vi "SQL Open.vi"(8 "error in (no error)":errorcluster, 11 "Ini Reference":T1) -> (0 "error out":errorcluster, 3 "SQL Address":string)   [LabVIEW 2012]
uses:
  <vilib>/Utility/config.llb/Config Data RefNum.ctl
  <vilib>/Utility/config.llb/Read Key (String).vi
  <vilib>/Utility/config.llb/NI_LVConfig.lvlib
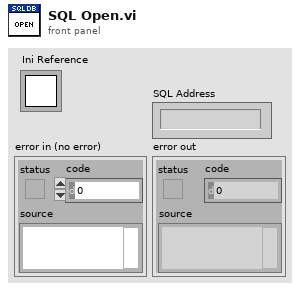
[diagram p1: front panel]
types:
  T1 = typedef "NI_LVConfig.lvlib/Config Data RefNum.ctl" = refnum<k1>
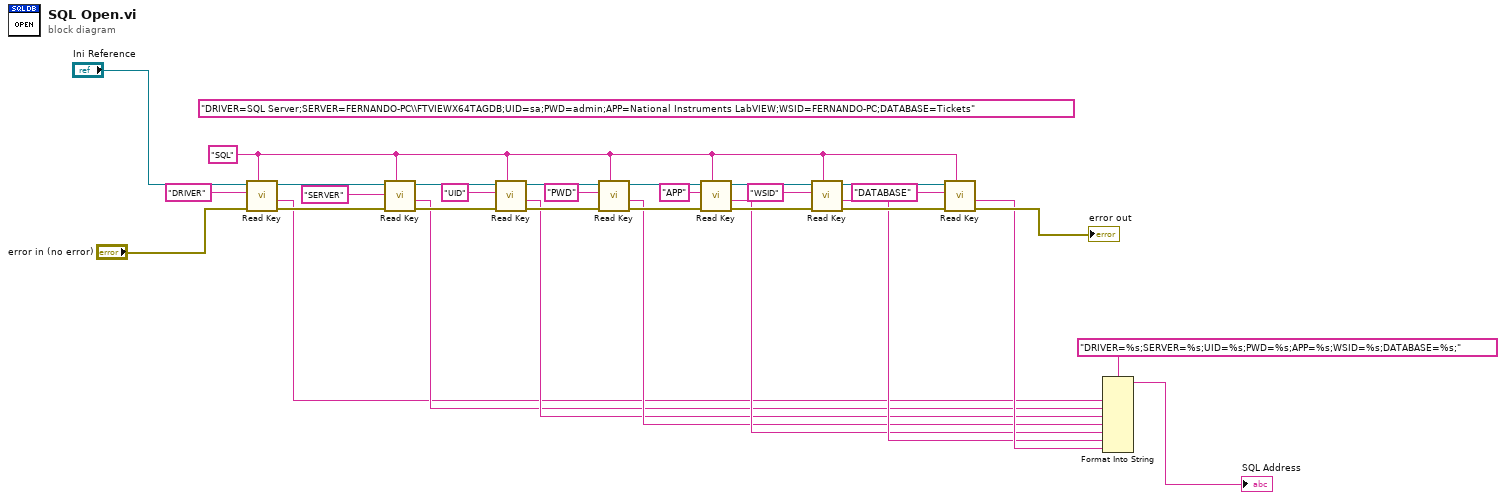
[diagram p0: block diagram]
diagram:
  (unwired) "DRIVER=SQL Server;SERVER=FERNANDO-PC\\FTVIEWX64TAGDB;UID=sa;PWD=admin;APP=National Instruments LabVIEW;WSID=FERNANDO-PC;DATABASE=Tickets"
  w32 = "SQL" ("section")
  n1 = call-poly <vilib>:"Read Key.vi"("section"=w32, "error in (no error)"="error in (no error)", "key"="DRIVER", "refnum"="Ini Reference") -> ("error out"=w14:errorcluster, "value"=w1:string, "refnum out"=w15:T1)  [unwired: 4 in, 1 out]
  n2 = call-poly <vilib>:"Read Key.vi"("section"=w32, "error in (no error)"=w14, "key"="SERVER", "refnum"=w15) -> ("error out"=w17:errorcluster, "value"=w2:string, "refnum out"=w18:T1)  [unwired: 4 in, 1 out]
  n3 = call-poly <vilib>:"Read Key.vi"("section"=w32, "error in (no error)"=w17, "key"="UID", "refnum"=w18) -> ("error out"=w20:errorcluster, "value"=w3:string, "refnum out"=w26:T1)  [unwired: 4 in, 1 out]
  n4 = call-poly <vilib>:"Read Key.vi"("section"=w32, "error in (no error)"=w20, "key"="PWD", "refnum"=w26) -> ("error out"=w21:errorcluster, "value"=w4:string, "refnum out"=w25:T1)  [unwired: 4 in, 1 out]
  n5 = call-poly <vilib>:"Read Key.vi"("section"=w32, "error in (no error)"=w21, "key"="APP", "refnum"=w25) -> ("error out"=w22:errorcluster, "value"=w5:string, "refnum out"=w28:T1)  [unwired: 4 in, 1 out]
  n6 = call-poly <vilib>:"Read Key.vi"("section"=w32, "error in (no error)"=w22, "key"="WSID", "refnum"=w28) -> ("error out"=w23:errorcluster, "value"=w6:string, "refnum out"=w30:T1)  [unwired: 4 in, 1 out]
  n7 = call-poly <vilib>:"Read Key.vi"("section"=w32, "error in (no error)"=w23, "key"="DATABASE", "refnum"=w30) -> ("error out"=→"error out":errorcluster, "value"=w7:string)  [unwired: 4 in, 2 out]
  n8 = Format Into String(format string="DRIVER=%s;SERVER=%s;UID=%s;PWD=%s;APP=%s;WSID=%s;DATABASE=%s;", w1, w2, w3, w4, w5, w6, w7) -> (resulting string=→"SQL Address":string)  [unwired: 2 in, 1 out]
